vi "Synchronize to Scan Engine.vi"(8 "error in (no error)":errorcluster) -> (0 "error out":errorcluster, 3 "scans since last call":u32)   [LabVIEW 2020]
doc: "Synchronizes execution timing to the scan period of the NI Scan Engine. This VI waits for each scan to complete and triggers subsequent code to execute once the scan engine has updated all values."
uses:
  <resource>/objmgr/ni.var.rc
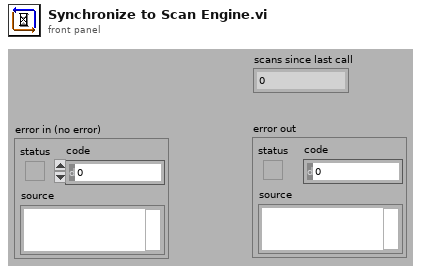
[diagram p1: front panel]
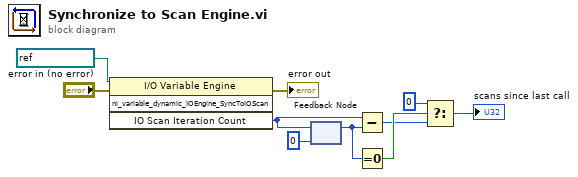
[diagram p0: block diagram]
diagram:
  n1 = invoke class="I/O Variable Engine" method="ni_variable_dynamic_IOEngine_SyncToIOScan"(reference=refnum<k21> "ni.var.io:/" ("reference out"), error in="error in (no error)") -> (error out=→"error out":errorcluster, "IO Scan Iteration Count"=w4:u64)  [unwired: 2 in, 2 out]
  n2 = feedback-in #1(w4) -> ()
  n3 = feedback #1(u64 0 ("IO Scan Iteration Count")) -> (w3:u64)
  n4 = Subtract(x=w4, y=w3) -> (x-y=w2:u32)
  n5 = Equal To 0?(x=w3) -> (x = 0?=w6:bool)
  n6 = Select(t=u32 0, s=w6, f=w2) -> (s? t:f=→"scans since last call":u32)
